vi "Assign CLT GPIO Pins.vi"(5 "Busy Pin (14: NONE)":i32(ring)=14 items=["EXT1", "EXT2", "EXT3", "EXT4", "EXT5", "EXT6", "EXT7", "EXT8", "EXT9", "EXT10", "EXT11", "EXT12", "EXT13", "EXT14", "NONE"], 6 "EOT Pin (14: NONE)":i32(ring)=14 items=["EXT1", "EXT2", "EXT3", "EXT4", "EXT5", "EXT6", "EXT7", "EXT8", "EXT9", "EXT10", "EXT11", "EXT12", "EXT13", "EXT14", "NONE"], 7 "SOT Pin (14: NONE)":i32(ring)=14 items=["EXT1", "EXT2", "EXT3", "EXT4", "EXT5", "EXT6", "EXT7", "EXT8", "EXT9", "EXT10", "EXT11", "EXT12", "EXT13", "EXT14", "NONE"], 8 "error in (no error)":errorcluster, 9 "Result Pins (Empty Array)":i32[](array[ring]) items=["EXT1", "EXT2", "EXT3", "EXT4", "EXT5", "EXT6", "EXT7", "EXT8", "EXT9", "EXT10", "EXT11", "EXT12", "EXT13", "EXT14"], 10 "Channel (0: Channel 1)":i32(ring) items=["Channel 1", "Channel 2"], 11 "VISA resource name":refnum<visa-resource-name>) -> (0 "error out":errorcluster, 3 "VISA resource name out":refnum<visa-resource-name>)   [LabVIEW 2023, in "Agilent B2900 Series.lvlib"]
doc: "Assigns the GPIO pins used for composite limit test and the result output.\n\n<B>Note:</B>\nThis VI is not applicable for Agilent models B2961A, B2962A, B2961B, B2962B, B2961C and B2962C."
uses:
  Agilent B2900 Series.lvlib
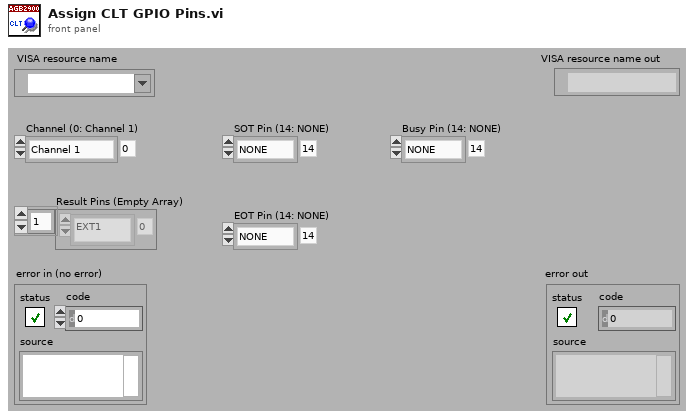
[diagram p1: front panel]
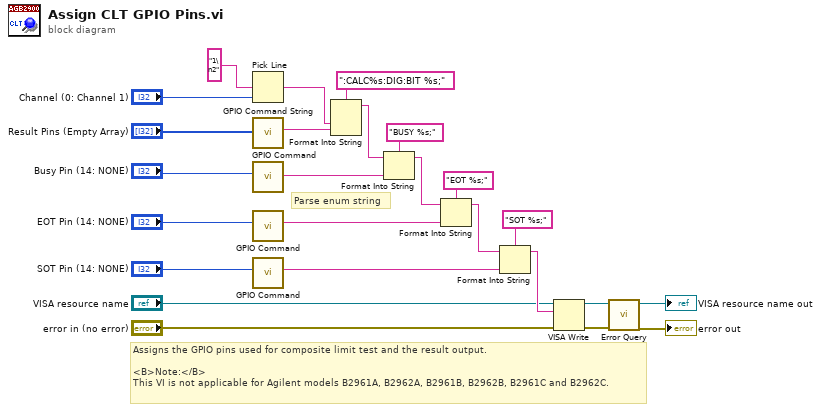
[diagram p0: block diagram]
diagram:
  # "Assigns the GPIO pins used for composite limit test and the result output.\n\n<B>Note:</B>\nThis VI is not applicable for Agilent models B2961A, B2962A, B2961B, B2962B, B2961C and B2962C."
  # "Parse enum string"
  n1 = Pick Line(multi-line string="1\n2" ("string (\"\")"), line index="Channel (0: Channel 1)") -> (output string=w7:string)  [unwired: 1 in]
  n2 = call "GPIO Command String.vi"("Pins For Result Output (Empty Array)"="Result Pins (Empty Array)") -> ("Result Command String"=w8:string)  [unwired: 10 in]
  n3 = call "GPIO Command.vi"("Pin(14: NONE)"="Busy Pin (14: NONE)") -> ("Command String"=w5:string)  [unwired: 10 in]
  n4 = call "GPIO Command.vi"("Pin(14: NONE)"="EOT Pin (14: NONE)") -> ("Command String"=w4:string)  [unwired: 10 in]
  n5 = call "GPIO Command.vi"("Pin(14: NONE)"="SOT Pin (14: NONE)") -> ("Command String"=w2:string)  [unwired: 10 in]
  n6 = Format Into String(format string=":CALC%s:DIG:BIT %s;", w7, w8) -> (resulting string=w24:string)  [unwired: 2 in, 1 out]
  n7 = Format Into String(format string="BUSY %s;", initial string=w24, w5) -> (resulting string=w22:string)  [unwired: 1 in, 1 out]
  n8 = Format Into String(format string="EOT %s;", initial string=w22, w4) -> (resulting string=w20:string)  [unwired: 1 in, 1 out]
  n9 = Format Into String(format string="SOT %s;", initial string=w20, w2) -> (resulting string=w18:string)  [unwired: 1 in, 1 out]
  n10 = VISA Write(VISA resource name="VISA resource name", write buffer=w18, error in (no error)="error in (no error)") -> (VISA resource name out=w15:refnum<visa-resource-name>, error out=w14:errorcluster)  [unwired: 1 out]
  n11 = call "Error Query.vi"("error in (no error)"=w14, "VISA resource name"=w15) -> ("error out"=→"error out":errorcluster, "VISA resource name out"=→"VISA resource name out":refnum<visa-resource-name>)  [unwired: 6 in, 2 out]
